vi "Export DataTable Columns.vi"(8 "error in (no error)":errorcluster, 11 "DataTable In":refnum<class "DataTable.lvclass">) -> (0 "error out":errorcluster, 2 "ColumnSetup":T1[](array[typedef]) {"MinWidth" min=2 step=1; "AutoSizeMode" items=["None"=1, "ColumnHeader"=2, "AllCellsExceptHeader"=4, "AllCells"=6, "DisplayedCellsExceptHeader"=8, "DisplayedCells"=10, "Fill"=16]; "FillWeight" min=1 max=100}, 3 "DataTable Out":refnum<class "DataTable.lvclass">)   [LabVIEW 2016, in "DataGrid.lvlib" / "DataTable.lvclass"]
doc: "Defines the columns of the dataTable that is used to store all display data. If called more than once, it will add columns to the existing dataTable, so resulting in more (possibly duplicate) columns."
uses:
  <userlib>/LabVIEWdotNetDataGrid/source/DataTable/DataTable.lvclass
  <userlib>/LabVIEWdotNetDataGrid/source/GridColumn/ColumnDefinition.ctl
  <userlib>/LabVIEWdotNetDataGrid/source/GridColumn/ColumnType.ctl
  <userlib>/LabVIEWdotNetDataGrid/source/DataTable/DataTable.lvclass/DataTable.ctl
  <userlib>/LabVIEWdotNetDataGrid/source/GridColumn/GridColumn.lvclass/GridColumn.ctl
  <userlib>/LabVIEWdotNetDataGrid/source/GridColumn/Read Name.vi
  <userlib>/LabVIEWdotNetDataGrid/source/GridColumn/Read Caption.vi
  <userlib>/LabVIEWdotNetDataGrid/source/GridColumn/Read datatype.vi
  <userlib>/LabVIEWdotNetDataGrid/source/GridColumn/Read Params.vi
  <userlib>/LabVIEWdotNetDataGrid/source/GridColumn/Read AutoSizeMode.vi
  <userlib>/LabVIEWdotNetDataGrid/source/GridColumn/Read FillWeight.vi
  <userlib>/LabVIEWdotNetDataGrid/source/GridColumn/Read Tooltip.vi
  <userlib>/LabVIEWdotNetDataGrid/source/GridColumn/Read ReadOnly.vi
  <userlib>/LabVIEWdotNetDataGrid/source/GridColumn/Read Visible.vi
  <userlib>/LabVIEWdotNetDataGrid/source/GridColumn/GridColumn.lvclass
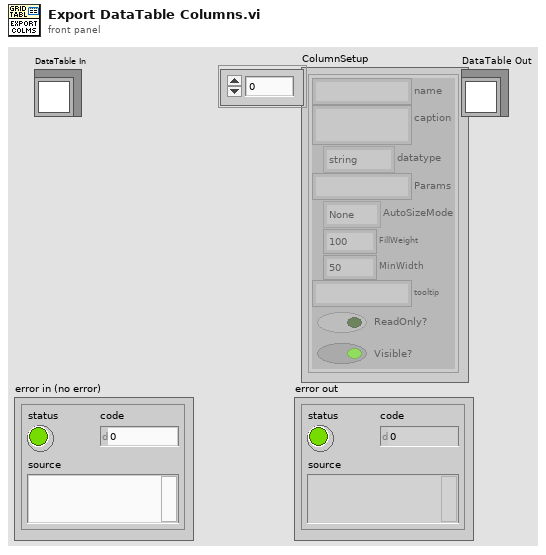
[diagram p1: front panel]
types:
  T1 = typedef "DataGrid.lvlib/GridColumn.lvclass/ColumnDefinition.ctl" = cluster{"name":string, "caption":string, "datatype":T2, "Params":string, "AutoSizeMode":i32, "FillWeight":sgl, "MinWidth":u32, "tooltip":string, "ReadOnly?":bool, "Visible?":bool}
  T2 = typedef "DataGrid.lvlib/GridColumn.lvclass/ColumnType.ctl" = enum16{"string", "image", "check", "numeric", "timestamp", "button", "combo", "link"}
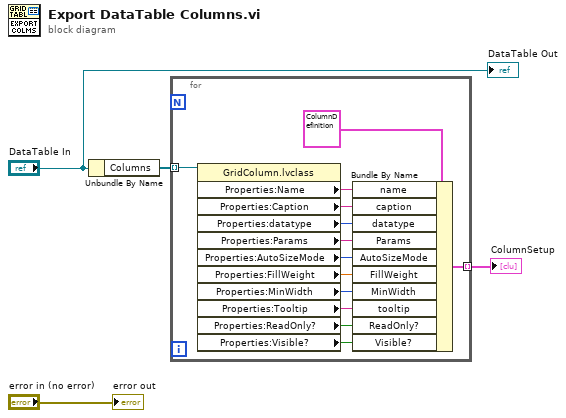
[diagram p0: block diagram]
diagram:
  n1 = Unbundle By Name("DataTable In") -> ("Columns"=w3:refnum<class "GridColumn.lvclass">[])
  n2 = for {
    tunnel: w3 -> [w17] mode=indexing
    tunnel: [w5] -> w2 mode=indexing
    n3 = property class="GridColumn.lvclass"(reference=w17) -> ("Properties:Name"=w15:string, "Properties:Caption"=w14:string, "Properties:datatype"=w13:T2, "Properties:Params"=w12:string, "Properties:AutoSizeMode"=w11:i32, "Properties:FillWeight"=w10:sgl, "Properties:MinWidth"=w9:i32, "Properties:Tooltip"=w8:string, "Properties:ReadOnly?"=w7:bool, "Properties:Visible?"=w6:bool)  [unwired: 1 in, 2 out]
    n4 = Bundle By Name(cluster=T1 {"name"="", "caption"="", "datatype"=enum."string", "Params"="", "AutoSizeMode"=1, "FillWeight"=100.0, "MinWidth"=50, "tooltip"="", "ReadOnly?"=FALSE, "Visible?"=TRUE} ("Column"), "name"=w15, "caption"=w14, "datatype"=w13, "Params"=w12, "AutoSizeMode"=w11, "FillWeight"=w10, "MinWidth"=w9, "tooltip"=w8, "ReadOnly?"=w7, "Visible?"=w6) -> (w5:T1)
  }
  "ColumnSetup" <- w2
  "error out" <- "error in (no error)"
  "DataTable Out" <- "DataTable In"
